vi "sns application sample.vi"() -> ()   [LabVIEW 2015]
uses:
  Core/HTTP Request/AWS Credentials.ctl
  Core/HTTP Request/Region.ctl
  Platform Application/Platform.ctl
  Platform Application/Application Attribute Value Pair.ctl
  Platform Application/Application Attribute.ctl
  Platform Application/Platform Application.lvclass
  Core/HTTP Request/HTTP Request.lvclass
panel:
  out "Array":string[](array[string])
  out "error out":errorcluster
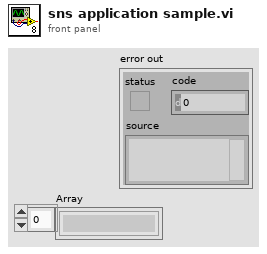
[diagram p1: front panel]
types:
  T1 = typedef "NI_AWS_SNS.lvlib/Platform Application.lvclass/Application Attribute Value Pair.ctl" = cluster{"Application attribute":T2, "Value":string}
  T2 = typedef "NI_AWS_SNS.lvlib/Platform Application.lvclass/Application Attribute.ctl" = enum16{"PlatformCredential", "PlatformPrincipal", "EventEndpointCreated", "EventEndpointDeleted", "EventEndpointUpdated", "EventDeliveryFailure", "SuccessFeedbackRoleArn", "FailureFeedbackRoleArn", "SuccessFeedbackSampleRate"}
  T3 = typedef "NI_AWS_SNS.lvlib/Platform Application.lvclass/Platform.ctl" = enum16{"ADM", "APNS", "APNS_SANDBOX", "GCM"}
  T4 = typedef "NI_AWS_Core.lvlib/HTTP Request.lvclass/Region.ctl" = enum16{"us-east-1", "us-east-2", "us-west-1", "us-west-2", "ap-northeast-1", "ap-northeast-2", "ap-southeast-1", "ap-southeast-2", "ca-central-1", "eu-central-1", "eu-west-1", "eu-west-2", "sa-east-1"}
  T5 = typedef "NI_AWS_Core.lvlib/HTTP Request.lvclass/AWS Credentials.ctl" = cluster{"Access Key":string, "Secret Key":string}
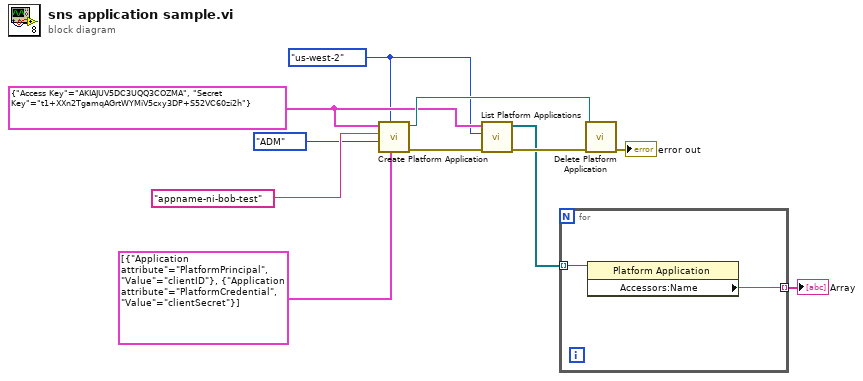
[diagram p0: block diagram]
diagram:
  w3 = Region."us-west-2" ("Region")
  w4 = T5 {"Access Key"="AKIAJUV5DC3UQQ3COZMA", "Secret Key"="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"} ("AWS Credentials")
  n1 = call "Create Platform Application.vi"("Platform Application Attributes"=T1[] [{"Application attribute"=enum."PlatformPrincipal", "Value"="clientID"}, {"Application attribute"=enum."PlatformCredential", "Value"="clientSecret"}], "Region"=w3, "Platform"=Platform."ADM", "Name"="appname-ni-bob-test", "AWS Credentials"=w4) -> ("error out"=w9:errorcluster, "Platform application out"=w5:refnum<class "Platform Application.lvclass">)  [unwired: 5 in]
  n2 = call "List Platform Applications.vi"("error in (no error)"=w9, "Region"=w3, "AWS Credentials"=w4) -> ("error out"=w6:errorcluster, "Platform Applications out"=w2:refnum<class "Platform Application.lvclass">[])  [unwired: 7 in]
  n3 = for {
    tunnel: w2 -> [w13] mode=indexing
    tunnel: [w12] -> w1 mode=indexing
    n4 = property class="Platform Application"(reference=w13) -> ("Accessors:Name"=w12:string)  [unwired: 1 in, 2 out]
  }
  "Array" <- w1
  n5 = call "Delete Platform Application.vi"("error in (no error)"=w6, "Platform Application in"=w5) -> ("error out"=→"error out":errorcluster)  [unwired: 9 in]
